vi "dispose connection.vi"(8 "error in":errorcluster, 11 "lvlibretls connection in":refnum<class "lvlibretls connection.lvclass">) -> (0 "error out":errorcluster, 3 "connection":refnum<k5>)   [LabVIEW 2016, in "lvlibretls connection.lvclass"]
doc: "dispose the connection object and return the original tcp connection for disposal (or continued use)"
uses:
  lvlibretls connection.lvclass
  lvlibretls connection.lvclass/lvlibretls connection.ctl
  lv tls dll.lvlib
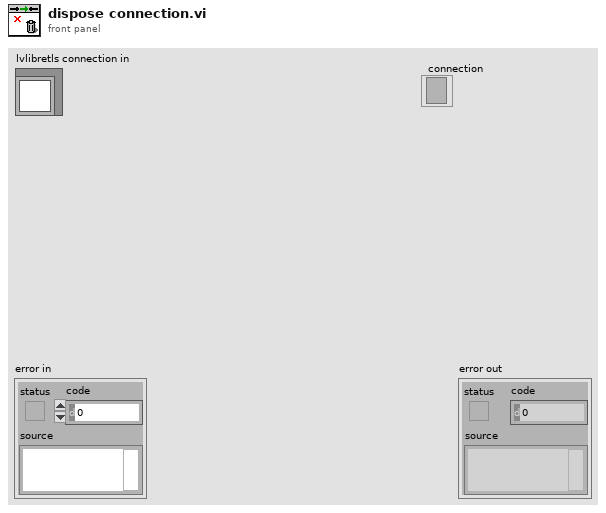
[diagram p1: front panel]
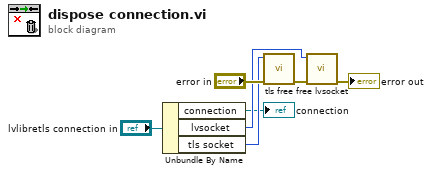
[diagram p0: block diagram]
diagram:
  n1 = Unbundle By Name("lvlibretls connection in") -> ("connection"=→"connection":refnum<k5>, "lvsocket"=w3:u64, "tls socket"=w2:u64)
  n2 = call "tls free.vi"("error in"="error in", "tls context"=w2) -> ("error out"=w6:errorcluster)  [unwired: 9 in]
  n3 = call "free lvsocket.vi"("error in"=w6, "lvsocket"=w3) -> ("error out"=→"error out":errorcluster)  [unwired: 9 in]
